vi "Get Size.vi"(8 "error in (no error)":errorcluster, 11 "Channel Configuration in":refnum<class "Configuration.Channel.lvclass">) -> (0 "error out":errorcluster, 2 "size in bytes":u64, 3 "Channel Configuration out":refnum<class "Configuration.Channel.lvclass">)   [LabVIEW 2016, in "Data Sharing Framework.Configuration.lvlib" / "Configuration.Channel.lvclass"]
uses:
  Configuration.Channel.lvclass
  Configuration.Channel.lvclass/Configuration.Channel.ctl
  <vilib>/NI Veristand/VeriStand Data/VeriStand Data.lvlib
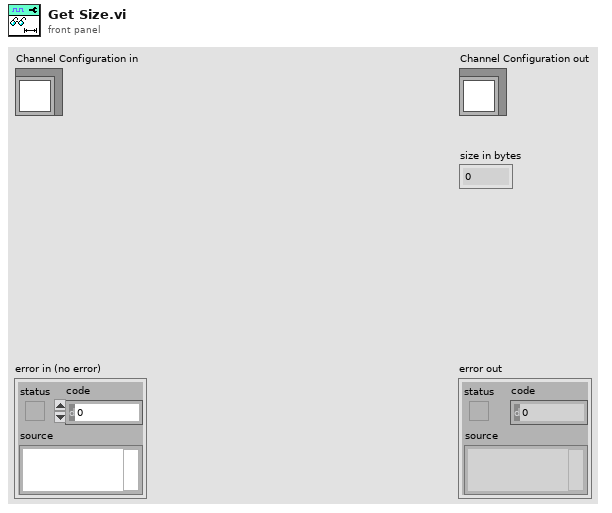
[diagram p1: front panel]
types:
  T1 = typedef "VeriStand Data.lvlib/Typedefs.Data Types.ctl" = enum16{"Boolean", "Single", "Double", "I8", "I16", "I32", "I64", "U8", "U16", "U32", "U64"}
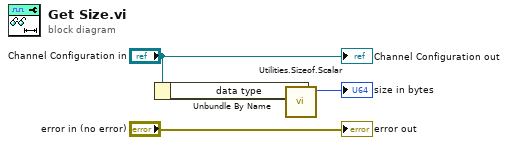
[diagram p0: block diagram]
diagram:
  n1 = Unbundle By Name("Channel Configuration in") -> ("data type"=w4:T1)
  n2 = call <vilib>:"Utilities.Sizeof.Scalar.vi"("data type"=w4) -> ("size in bytes"=→"size in bytes":u64)  [unwired: 9 in, 1 out]
  "error out" <- "error in (no error)"
  "Channel Configuration out" <- "Channel Configuration in"
